vi "CalculateBand.vi"(0 "waveform":waveform(sgl), 1 "channel name of waveform to use in phase band calculation":string, 2 "conversion op":T1, 3 "waveform to use in phase band calculation":waveform(sgl), 5 "speed [RPM]":dbl, 7 "feature":T2, 9 "pulse positions":dbl[](array[numeric]), 11 "error in (no error)":errorcluster, 12 "calc cache":variant) -> (6 "band value":dbl, 14 "calc cache out":variant, 15 "error out":errorcluster)   [LabVIEW 2017, in "AnalysisHelper.lvlib"]
uses:
  <vilib>/addons/InsightCM/Utilities/Analysis/Shared/AnalysisHelper.lvlib
  <vilib>/addons/InsightCM/Utilities/Analysis/Shared/controls/Feature.ctl
  <vilib>/addons/InsightCM/Utilities/Analysis/Shared/controls/AmplitudeScale.ctl
  <vilib>/addons/InsightCM/Utilities/Analysis/Shared/controls/ConversionOp.ctl
  <vilib>/addons/InsightCM/Utilities/Analysis/Shared/controls/BandConfig.ctl
  <vilib>/addons/InsightCM/Utilities/Analysis/Shared/controls/BandDomain.ctl
  <vilib>/addons/InsightCM/Utilities/Analysis/Shared/controls/BandCalculation.ctl
  <vilib>/Analysis/coordinate.llb/Angle Units.ctl
  <vilib>/Analysis/coordinate.llb/Angle Range (Degree).ctl
  <vilib>/Analysis/coordinate.llb/Wrap Angle (scalar).vi
  <vilib>/addons/InsightCM/Utilities/Analysis/Vibration/subVIs/Band Magnitude - Total (Frequency).vi
  <vilib>/addons/InsightCM/Utilities/Analysis/Vibration/subVIs/Band Magnitude - Peak (Frequency).vi
  <vilib>/addons/InsightCM/Utilities/Analysis/Vibration/subVIs/Band Magnitude - Total (CPM).vi
  <vilib>/addons/InsightCM/Utilities/Analysis/Vibration/subVIs/Band Magnitude - Peak (CPM).vi
  <vilib>/addons/InsightCM/Utilities/Analysis/Vibration/subVIs/Band Magnitude - Total (Orders).vi
  <vilib>/addons/InsightCM/Utilities/Analysis/Vibration/subVIs/Band Magnitude - Peak (Orders).vi
  <vilib>/addons/InsightCM/Utilities/Analysis/Vibration/subVIs/Band Phase (Frequency).vi
  <vilib>/addons/InsightCM/Utilities/Analysis/Vibration/subVIs/Band Phase (CPM).vi
  <vilib>/addons/InsightCM/Utilities/Analysis/Vibration/subVIs/Band Phase (Orders).vi
  <vilib>/addons/InsightCM/Utilities/Analysis/Vibration/VibrationAnalysisFunctions.lvlib
  <vilib>/Analysis/NI_AAL_Angle.lvlib
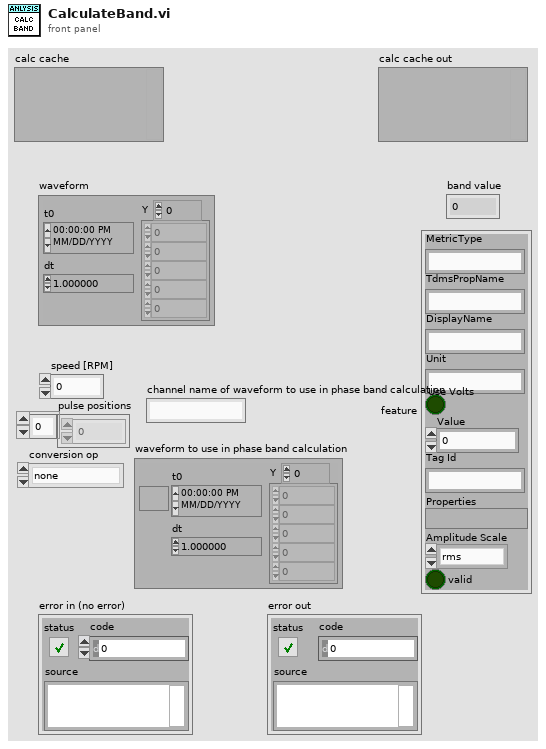
[diagram p1: front panel]
types:
  T1 = typedef "AnalysisHelper.lvlib/ConversionOp.ctl" = enum16{"none", "singleInt", "doubleInt", "singleDiff", "doubleDiff"}
  T2 = typedef "AnalysisHelper.lvlib/Feature.ctl" = cluster{"MetricType":string, "TdmsPropName":string, "DisplayName":string, "Unit":string, "Use Volts":bool, "Value":dbl, "Tag Id":string, "Properties":variant, "Amplitude Scale":T3, "valid":bool}
  T3 = typedef "AnalysisHelper.lvlib/AmplitudeScale.ctl" = enum16{"rms", "peak", "pk-pk"}
  T4 = typedef "AnalysisHelper.lvlib/BandConfig.ctl" = cluster{"High":dbl, "Low":dbl, "Domain":T5, "Calculation":T6}
  T5 = typedef "AnalysisHelper.lvlib/BandDomain.ctl" = enum16{"Frequency", "CPM", "Orders"}
  T6 = typedef "AnalysisHelper.lvlib/BandCalculation.ctl" = enum16{"Total", "Max", "Phase"}
  T7 = typedef "svc_Spectrum Info.ctl" = cluster{"channel name":string, "description":string, "x-axis units":T8, "spectral info":cluster{"spectrum type":T9, "linear/dB":enum16{"linear", "dB"}, "window":u16, "window size":i32, "FFT size":i32}, "engineering units":T10, "custom label":string, "dB reference [EU]":dbl, "peak units":enum16{"rms", "peak", "peak-peak"}, "weighting filter":T11, "spectral density?":bool, "unit label":string, "spectrum skewed?":bool, "complimentary spectrum units":T12}
  T8 = typedef "svc_X-Axis Units.ctl" = u16
  T9 = typedef "svc_Spectrum Type.ctl" = enum16{"FFT Spectrum [complex]", "Amplitude [Magnitude]", "Power [Magnitude^2]", "Cross Spectrum [complex]", "Frequency Response [Complex]"}
  T10 = typedef "svc_Engineering Units Text Ring.ctl" = u16
  T11 = typedef "svc_Weighting Filter Text Ring.ctl" = u16
  T12 = typedef "svc_Complimentary Spectrum Units.ctl" = enum16{"none", "radians", "degrees", "cycles", "imaginary"}
  T13 = typedef "NI_AAL_Angle.lvlib/Angle Range (Degree).ctl" = u16
  T14 = typedef "NI_AAL_Angle.lvlib/Angle Units.ctl" = i32
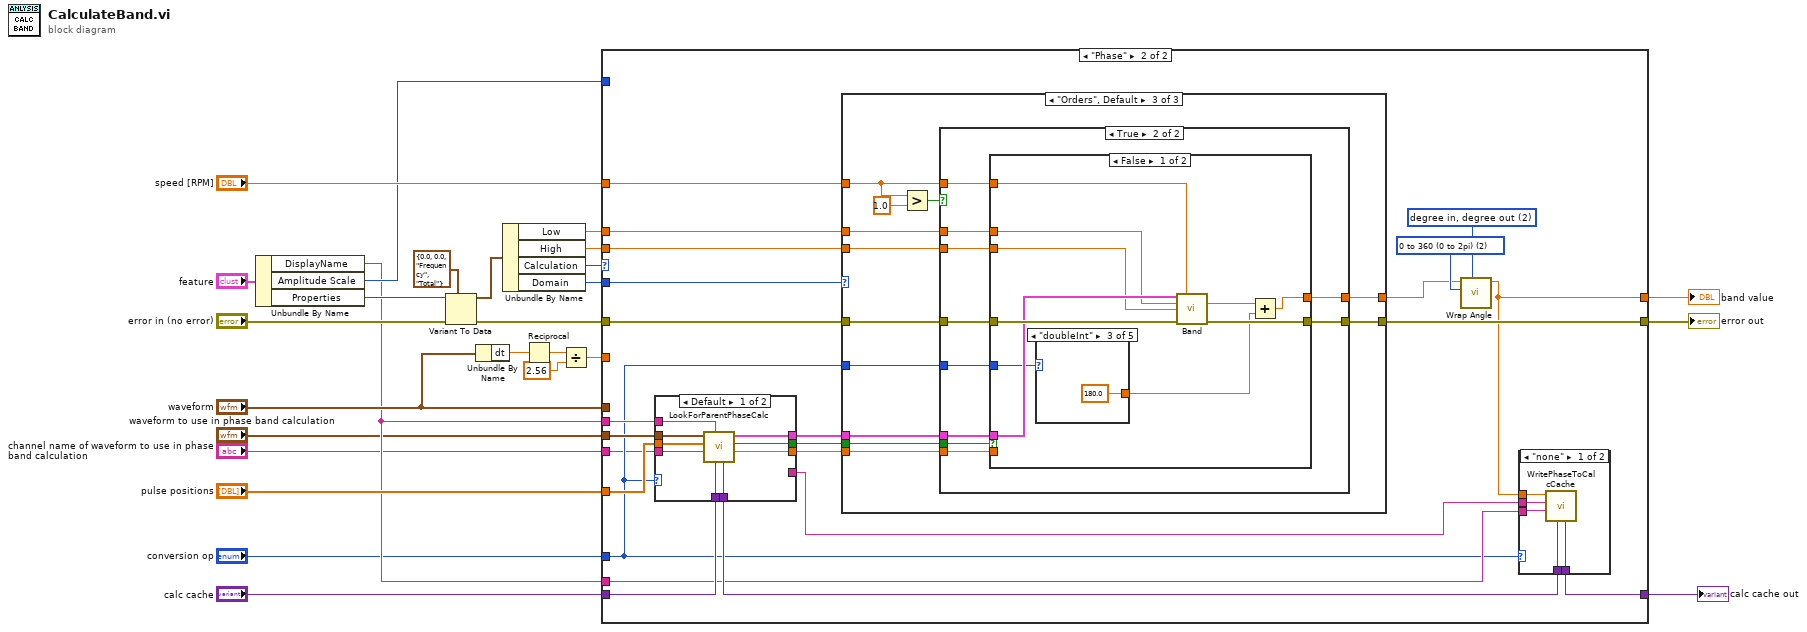
[diagram p0: block diagram]
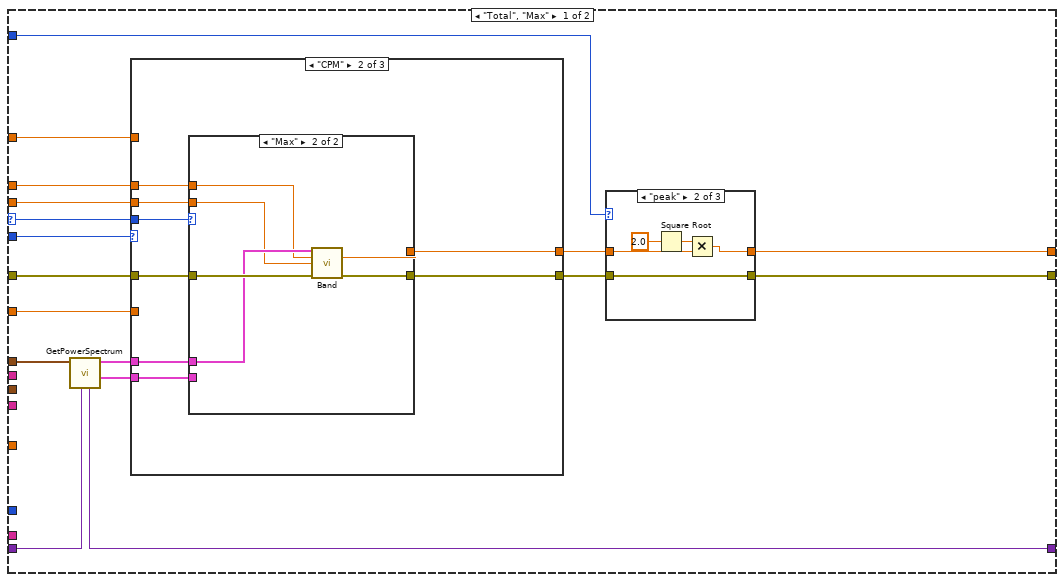
[diagram p2: hidden frame]
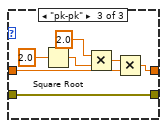
[diagram p4: hidden frame]
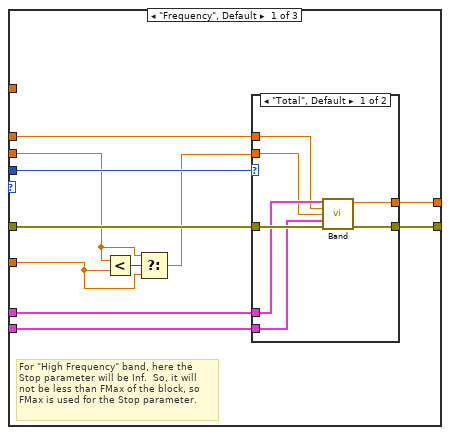
[diagram p5: hidden frame]
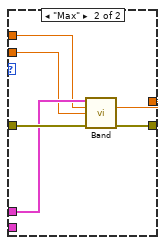
[diagram p6: hidden frame]
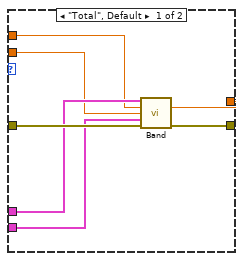
[diagram p7: hidden frame]
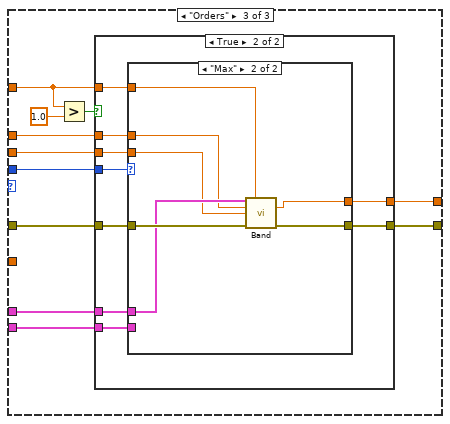
[diagram p8: hidden frame]
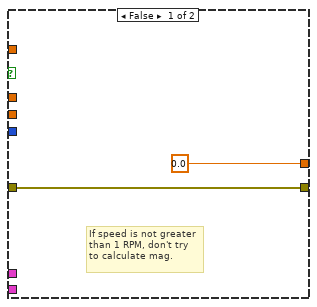
[diagram p9: hidden frame]
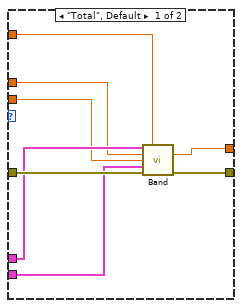
[diagram p10: hidden frame]
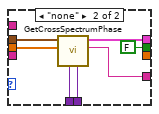
[diagram p12: hidden frame]
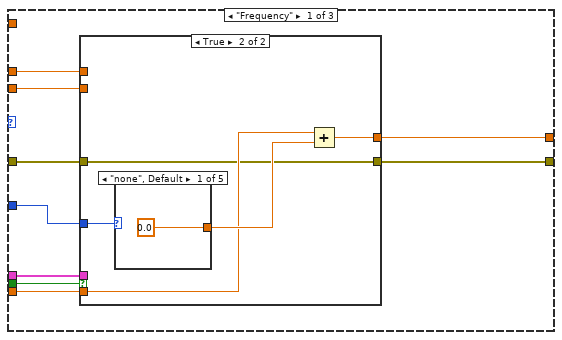
[diagram p13: hidden frame]
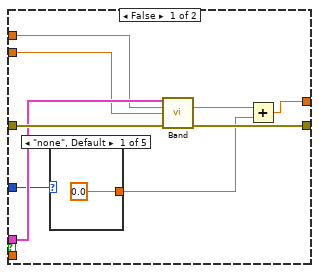
[diagram p14: hidden frame]
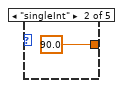
[diagram p15: hidden frame]
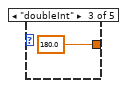
[diagram p16: hidden frame]
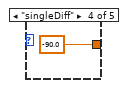
[diagram p17: hidden frame]
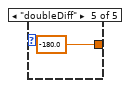
[diagram p18: hidden frame]
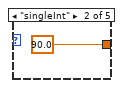
[diagram p19: hidden frame]
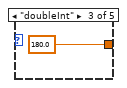
[diagram p20: hidden frame]
diagram:
  n1 = Unbundle By Name("feature") -> ("DisplayName"=w4:string, "Amplitude Scale"=w8:T3, "Properties"=w10:variant)
  n2 = Variant To Data(error in="error in (no error)", type=T4 {"High"=0.0, "Low"=0.0, "Domain"=enum."Frequency", "Calculation"=enum."Total"} ("SpectralBand"), Variant=w10) -> (data=w16:T4, error out=w18:errorcluster)
  n3 = Unbundle By Name("waveform") -> ("dt"=w20:dbl)
  n4 = Unbundle By Name(w16) -> ("Low"=w15:dbl, "High"=w14:dbl, "Calculation"=w13:T6, "Domain"=w12:T5)
  n5 = Reciprocal(x=w20) -> (1/x=w21:dbl)
  n6 = Divide(x=w21, y=2.56) -> (x/y=w22:dbl)
  n7 = case shown="\"Phase\"" w13 {
    selector: w13 -> [w35 _]
    tunnel: w18 -> [w43 w140]
    tunnel: w12 -> [w42 w162]
    tunnel: "speed [RPM]" -> [w41 w161]
    tunnel: [w29 w151] -> w25
    tunnel: [w33 w160] -> w24
    tunnel: w14 -> [w40 w159]
    tunnel: w15 -> [w39 w158]
    tunnel: "waveform" -> [w36 _]
    tunnel: "pulse positions" -> [_ w153]
    tunnel: w22 -> [w34 _]
    tunnel: w8 -> [w30 _]
    tunnel: "calc cache" -> [w28 w152]
    tunnel: [w27 w149] -> w5
    tunnel: w4 -> [_ w147]
    tunnel: w4 -> [_ w146]
    tunnel: "waveform to use in phase band calculation" -> [_ w143]
    tunnel: "conversion op" -> [_ w142]
    tunnel: "channel name of waveform to use in phase band calculation" -> [_ w141]
    frame "Total", "Max" {
      n8 = call <vilib>:"GetPowerSpectrum.vi"("calc cache"=w28, "Waveform"=w36) -> ("spectrum info"=w37:T7, "power spectrum [EU^2 rms]"=w38:cluster{"f0":dbl, "df":dbl, "magnitude":sgl[]}, "calc cache out"=w27:variant)  [unwired: 7 in]
      n9 = case shown="\"CPM\"" w42 {
        tunnel: w43 -> [w68 w89 w113]
        tunnel: [w65 w88 w112] -> w32
        tunnel: w38 -> [w62 w86 w111]
        tunnel: w37 -> [w67 w85 w110]
        tunnel: [w66 w87 w106] -> w31
        tunnel: w41 -> [_ _ w108]
        tunnel: w40 -> [w60 w83 w105]
        tunnel: w39 -> [w64 w84 w104]
        tunnel: w35 -> [w63 w82 w103]
        tunnel: w34 -> [w58 _ _]
        frame "Frequency", Default {
          # "For \"High Frequency\" band, here the\nStop parameter will be Inf.  So, it will\nnot be less than FMax of the block, so\nFMax is used for the Stop parameter."
          n10 = Less?(x=w60, y=w58) -> (x < y?=w61:bool)
          n11 = Select(t=w60, s=w61, f=w58) -> (s? t:f=w59:dbl)
          n12 = case shown="\"Total\", Default" w63 {
            tunnel: w68 -> [w75 w81]
            tunnel: w62 -> [w74 w80]
            tunnel: w67 -> [w73 _]
            tunnel: [w72 w79] -> w66
            tunnel: [w71 w78] -> w65
            tunnel: w64 -> [w70 w77]
            tunnel: w59 -> [w69 w76]
            frame "Total", Default {
              n13 = call-poly <vilib>:"Band.vi"("power spectrum [EU^2 rms]"=w74, "Start"=w70, "Stop"=w69, "spectrum info"=w73, "error in (no error)"=w75) -> ("Total Magnitude [EU rms]"=w72:sgl, "error out"=w71:errorcluster)  [unwired: 9 in]
            }
            frame "Max" {
              n14 = call-poly <vilib>:"Band.vi"("power spectrum [EU^2 rms]"=w80, "Start"=w77, "Stop"=w76, "error in (no error)"=w81) -> ("Max Peak in Band [EU rms]"=w79:sgl, "error out"=w78:errorcluster)  [unwired: 10 in]
            }
          }
        }
        frame "CPM" {
          n15 = case shown="\"Max\"" w82 {
            tunnel: w89 -> [w96 w102]
            tunnel: [w95 w101] -> w88
            tunnel: [w94 w100] -> w87
            tunnel: w86 -> [w93 w99]
            tunnel: w85 -> [w92 _]
            tunnel: w84 -> [w91 w98]
            tunnel: w83 -> [w90 w97]
            frame "Total", Default {
              n16 = call-poly <vilib>:"Band.vi"("power spectrum [EU^2 rms]"=w93, "Start"=w91, "Stop"=w90, "spectrum info"=w92, "error in (no error)"=w96) -> ("total magnitude [EU rms]"=w94:sgl, "error out"=w95:errorcluster)  [unwired: 9 in]
            }
            frame "Max" {
              n17 = call-poly <vilib>:"Band.vi"("power spectrum [EU^2 rms]"=w99, "Start"=w98, "Stop"=w97, "error in (no error)"=w102) -> ("Max Peak In Band [EU rms]"=w100:sgl, "error out"=w101:errorcluster)  [unwired: 10 in]
            }
          }
        }
        frame "Orders" {
          n18 = Greater?(x=w108, y=sgl 1.0) -> (0:w107:bool)
          n19 = case shown="True" w107 {
            tunnel: w113 -> [w115 w124]
            tunnel: [w115 w119] -> w112
            tunnel: w111 -> [_ w123]
            tunnel: w110 -> [_ w122]
            tunnel: w108 -> [_ w121]
            tunnel: [sgl 0.0 ("Power in Band [EU^2 rms]") w120] -> w106
            tunnel: w105 -> [_ w118]
            tunnel: w104 -> [_ w117]
            tunnel: w103 -> [_ w116]
            frame False {
              # "If speed is not greater\nthan 1 RPM, don't try\nto calculate mag."
            }
            frame True {
              n20 = case shown="\"Max\"" w116 {
                tunnel: w124 -> [w132 w139]
                tunnel: w123 -> [w131 w138]
                tunnel: w122 -> [w130 _]
                tunnel: w121 -> [w129 w137]
                tunnel: [w128 w136] -> w120
                tunnel: [w127 w135] -> w119
                tunnel: w118 -> [w126 w134]
                tunnel: w117 -> [w125 w133]
                frame "Total", Default {
                  n21 = call-poly <vilib>:"Band.vi"("power spectrum [EU^2 rms]"=w131, "Speed (RPM)"=w129, "Start"=w125, "Stop"=w126, "spectrum info"=w130, "error in (no error)"=w132) -> ("Total Magnitude [EU rms]"=w128:sgl, "error out"=w127:errorcluster)  [unwired: 8 in]
                }
                frame "Max" {
                  n22 = call-poly <vilib>:"Band.vi"("power spectrum [EU^2 rms]"=w138, "Speed (RPM)"=w137, "Start"=w133, "Stop"=w134, "error in (no error)"=w139) -> ("Max Peak in Band [EU rms]"=w136:sgl, "error out"=w135:errorcluster)  [unwired: 9 in]
                }
              }
            }
          }
        }
      }
      n23 = case shown="\"peak\"" w30 {
        tunnel: [w44 w50 w57] -> w33
        tunnel: w32 -> [w44 w50 w57]
        tunnel: w31 -> [w45 w49 w56]
        tunnel: [w45 w48 w55] -> w29
        frame "rms", Default {
        }
        frame "peak" {
          n24 = Square Root(x=2.0) -> (sqrt(x)=w47:dbl)
          n25 = Multiply(x=w47, y=w49) -> (x*y=w48:dbl)
        }
        frame "pk-pk" {
          n26 = Square Root(x=2.0) -> (sqrt(x)=w52:dbl)
          n27 = Multiply(x=2.0, y=w52) -> (x*y=w53:dbl)
          n28 = Multiply(x=w53, y=w56) -> (x*y=w55:dbl)
        }
      }
    }
    frame "Phase" {
      w156 = T13 2 items=["none", "-180 to 180 (-pi to pi)", "0 to 360 (0 to 2pi)"] ("angle range")
      w157 = T14 2 items=["radian in, radian out", "radian in, degree out", "degree in, degree out", "degree in, radian out"] ("angle units")
      n29 = case shown="Default" w142 {
        tunnel: [w175 w184] -> w154
        tunnel: [w173 w183] -> w150
        tunnel: w152 -> [w174 w182]
        tunnel: w153 -> [w176 w181]
        tunnel: w143 -> [w177 w180]
        tunnel: [_ w179] -> w148
        tunnel: w141 -> [w169 _]
        tunnel: w147 -> [w170 _]
        tunnel: [w172 FALSE ("found cached parent phase")] -> w145
        tunnel: [w171 _] -> w144
        frame Default {
          n30 = call <vilib>:"LookForParentPhaseCalc.vi"("calc cache in"=w174, "feature name"=w170, "channel name"=w169, "pulse positions"=w176, "waveform to use in phase band calculation"=w177) -> ("parent channel phase value"=w171:dbl, "found cached parent phase"=w172:bool, "Cross phase [degrees]"=w175:cluster{"f0":dbl, "df":dbl, "phase":sgl[]}, "calc cache out"=w173:variant)  [unwired: 3 in]
        }
        frame "none" {
          n31 = call <vilib>:"GetCrossSpectrumPhase.vi"("calc cache"=w182, "speed profile (positions [s])"=w181, "waveform"=w180) -> ("channel name"=w179:string, "cross phase [degrees]"=w184:cluster{"f0":dbl, "df":dbl, "phase":sgl[]}, "calc cache out"=w183:variant)  [unwired: 5 in, 1 out]
        }
      }
      n32 = case shown="\"Orders\", Default" w162 {
        tunnel: w140 -> [w193 w226 w262]
        tunnel: [w191 w225 w261] -> w160
        tunnel: w154 -> [w192 w224 w260]
        tunnel: [w187 w220 w256] -> w155
        tunnel: w161 -> [_ _ w258]
        tunnel: w159 -> [w189 w222 w255]
        tunnel: w158 -> [w190 w223 w254]
        tunnel: w142 -> [w188 w221 w253]
        tunnel: w145 -> [w186 w219 w252]
        tunnel: w144 -> [w185 w218 w251]
        frame "Frequency" {
          n33 = case shown="True" w186 {
            tunnel: w193 -> [w202 w208]
            tunnel: w192 -> [w201 _]
            tunnel: [w200 w208] -> w191
            tunnel: w190 -> [w199 _]
            tunnel: w189 -> [w198 _]
            tunnel: w188 -> [w197 w212]
            tunnel: [w196 w211] -> w187
            tunnel: w185 -> [_ w209]
            frame False {
              n34 = case shown="\"none\", Default" w197 {
                tunnel: [sgl 0.0 ("y") sgl 90.0 ("y") sgl 180.0 ("y") sgl -90.0 ("y") sgl -180.0 ("y")] -> w194
                frame "none", Default {
                }
                frame "singleInt" {
                }
                frame "doubleInt" {
                }
                frame "singleDiff" {
                }
                frame "doubleDiff" {
                }
              }
              n35 = call-poly <vilib>:"Band.vi"("Cross phase [degrees]"=w201, "Start"=w199, "Stop"=w198, "error in (no error)"=w202) -> ("Phase (deg)"=w195:sgl, "error out"=w200:errorcluster)  [unwired: 10 in]
              n36 = Add(x=w195, y=w194) -> (x+y=w196:sgl)
            }
            frame True {
              n37 = case shown="\"none\", Default" w212 {
                tunnel: [sgl 0.0 ("y") sgl 90.0 ("y") sgl 180.0 ("y") sgl -90.0 ("y") sgl -180.0 ("y")] -> w210
                frame "none", Default {
                }
                frame "singleInt" {
                }
                frame "doubleInt" {
                }
                frame "singleDiff" {
                }
                frame "doubleDiff" {
                }
              }
              n38 = Add(x=w209, y=w210) -> (x+y=w211:dbl)
            }
          }
        }
        frame "CPM" {
          n39 = case shown="False" w219 {
            tunnel: w226 -> [w227 w245]
            tunnel: [w227 w244] -> w225
            tunnel: w224 -> [_ w243]
            tunnel: w223 -> [_ w242]
            tunnel: w222 -> [_ w241]
            tunnel: w221 -> [w231 w240]
            tunnel: [w230 w239] -> w220
            tunnel: w218 -> [w228 _]
            frame True {
              n40 = case shown="\"none\", Default" w231 {
                tunnel: [sgl 0.0 ("y") sgl 90.0 ("y") sgl 180.0 ("y") sgl -90.0 ("y") sgl -180.0 ("y")] -> w229
                frame "none", Default {
                }
                frame "singleInt" {
                }
                frame "doubleInt" {
                }
                frame "singleDiff" {
                }
                frame "doubleDiff" {
                }
              }
              n41 = Add(x=w228, y=w229) -> (x+y=w230:dbl)
            }
            frame False {
              n42 = case shown="\"none\", Default" w240 {
                tunnel: [sgl 0.0 ("y") sgl 90.0 ("y") sgl 180.0 ("y") sgl -90.0 ("y") sgl -180.0 ("y")] -> w237
                frame "none", Default {
                }
                frame "singleInt" {
                }
                frame "doubleInt" {
                }
                frame "singleDiff" {
                }
                frame "doubleDiff" {
                }
              }
              n43 = call-poly <vilib>:"Band.vi"("Cross phase [degrees]"=w243, "Start"=w242, "Stop"=w241, "error in (no error)"=w245) -> ("Phase (deg)"=w238:sgl, "error out"=w244:errorcluster)  [unwired: 10 in]
              n44 = Add(x=w238, y=w237) -> (x+y=w239:sgl)
            }
          }
        }
        frame "Orders", Default {
          n45 = Greater?(x=w258, y=sgl 1.0) -> (0:w257:bool)
          n46 = case shown="True" w257 {
            tunnel: w262 -> [w264 w274]
            tunnel: [w264 w271] -> w261
            tunnel: w260 -> [_ w273]
            tunnel: w258 -> [_ w272]
            tunnel: [sgl 0.0 ("Power in Band [EU^2 rms]") w268] -> w256
            tunnel: w255 -> [_ w270]
            tunnel: w254 -> [_ w269]
            tunnel: w253 -> [_ w267]
            tunnel: w252 -> [_ w266]
            tunnel: w251 -> [_ w265]
            frame False {
              # "If speed is not greater\nthan 1 RPM, don't try\nto calculate mag."
            }
            frame True {
              n47 = case shown="False" w266 {
                tunnel: w274 -> [w284 w290]
                tunnel: w273 -> [w283 _]
                tunnel: w272 -> [w282 _]
                tunnel: [w281 w290] -> w271
                tunnel: w270 -> [w280 _]
                tunnel: w269 -> [w279 _]
                tunnel: [w276 w293] -> w268
                tunnel: w267 -> [w275 w292]
                tunnel: w265 -> [_ w291]
                frame False {
                  n48 = case shown="\"doubleInt\"" w275 {
                    tunnel: [sgl 0.0 ("y") sgl 90.0 ("y") sgl 180.0 ("y") sgl -90.0 ("y") sgl -180.0 ("y")] -> w277
                    frame "none", Default {
                    }
                    frame "singleInt" {
                    }
                    frame "doubleInt" {
                    }
                    frame "singleDiff" {
                    }
                    frame "doubleDiff" {
                    }
                  }
                  n49 = call-poly <vilib>:"Band.vi"("Cross phase [degrees]"=w283, "Speed (RPM)"=w282, "Start"=w279, "Stop"=w280, "error in (no error)"=w284) -> ("Phase (deg)"=w278:sgl, "error out"=w281:errorcluster)  [unwired: 9 in]
                  n50 = Add(x=w278, y=w277) -> (x+y=w276:sgl)
                }
                frame True {
                  n51 = case shown="\"none\", Default" w292 {
                    tunnel: [sgl 0.0 ("y") sgl 90.0 ("y") sgl 180.0 ("y") sgl -90.0 ("y") sgl -180.0 ("y")] -> w294
                    frame "none", Default {
                    }
                    frame "singleInt" {
                    }
                    frame "doubleInt" {
                    }
                    frame "singleDiff" {
                    }
                    frame "doubleDiff" {
                    }
                  }
                  n52 = Add(x=w291, y=w294) -> (x+y=w293:dbl)
                }
              }
            }
          }
        }
      }
      n53 = call-poly <vilib>:"Wrap Angle.vi"("angle units"=w157, "angle range"=w156, "angle in"=w155) -> ("angle out"=w151:dbl)  [unwired: 7 in, 1 out]
      n54 = case shown="\"none\"" w142 {
        tunnel: w151 -> [w167 _]
        tunnel: w150 -> [w166 w168]
        tunnel: [w165 w168] -> w149
        tunnel: w148 -> [w164 _]
        tunnel: w146 -> [w163 _]
        frame "none" {
          n55 = call <vilib>:"WritePhaseToCalcCache.vi"("calc cache"=w166, "feature name"=w163, "channel name"=w164, "phase"=w167) -> ("calc cache out"=w165:variant)  [unwired: 7 in]
        }
        frame Default {
        }
      }
    }
  }
  "error out" <- w24
  "band value" <- w25
  "calc cache out" <- w5
